vi "Indent Size.vi"() -> (1 "indent":string, 3 "indent size":i32)   [LabVIEW 2020, in "infolib.lvlib"]
doc: "Returns number of spaces of set indent. Also creates a string of spaces of set indent. Indent is set in conditional symbols in project settings."
uses:
  infolib.lvlib
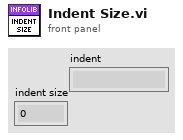
[diagram p1: front panel]
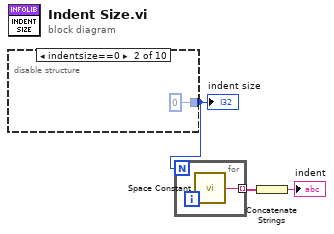
[diagram p0: block diagram]
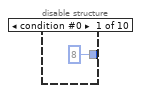
[diagram p2: hidden frame]
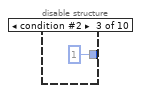
[diagram p3: hidden frame]
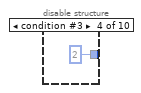
[diagram p4: hidden frame]
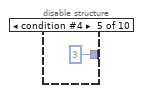
[diagram p5: hidden frame]
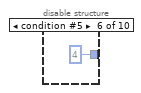
[diagram p6: hidden frame]
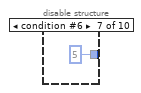
[diagram p7: hidden frame]
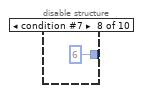
[diagram p8: hidden frame]
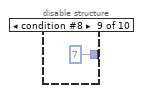
[diagram p9: hidden frame]
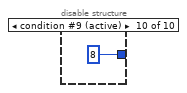
[diagram p10: hidden frame]
diagram:
  n1 = disable-structure shown="indentsize==0" {
    disable-tunnel: [8 ("spaces no") 0 ("spaces no") 1 ("spaces no") 2 ("spaces no") 3 ("spaces no") 4 ("spaces no") 5 ("spaces no") 6 ("spaces no") 7 ("spaces no") 8 ("spaces no")] -> w3
    frame condition #0 {
    }
    frame condition #1 {
    }
    frame condition #2 {
    }
    frame condition #3 {
    }
    frame condition #4 {
    }
    frame condition #5 {
    }
    frame condition #6 {
    }
    frame condition #7 {
    }
    frame condition #8 {
    }
    frame condition #9 (active) {
    }
  }
  "indent size" <- w3
  n2 = for {
    N: w3 -> [_]
    tunnel: [w14] -> w2 mode=indexing
    n3 = call <vilib>:"Space Constant.vi"() -> ("String"=w14:string)
  }
  n4 = Concatenate Strings(w2) -> (→"indent":string)
